vi "applyNewTimes.vi"(8 "error in (no error)":errorcluster, 11 "ScriptEventList in":refnum<class "ScriptEventList.lvclass">) -> (0 "error out":errorcluster, 3 "ScriptEventList out":refnum<class "ScriptEventList.lvclass">)   [LabVIEW 2011, in "Tools.lvlib" / "Scripting.lvlib" / "ScriptEventList.lvclass"]
uses:
  ScriptEventList.lvclass
  ScriptEventList.lvclass/ScriptEventList.ctl
  ScriptEvent.lvclass
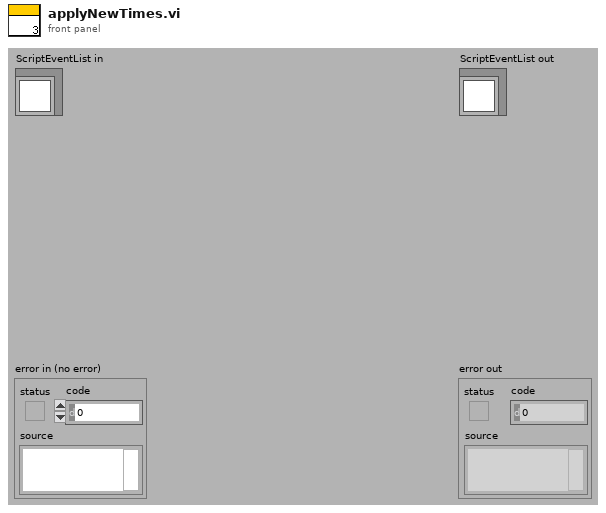
[diagram p1: front panel]
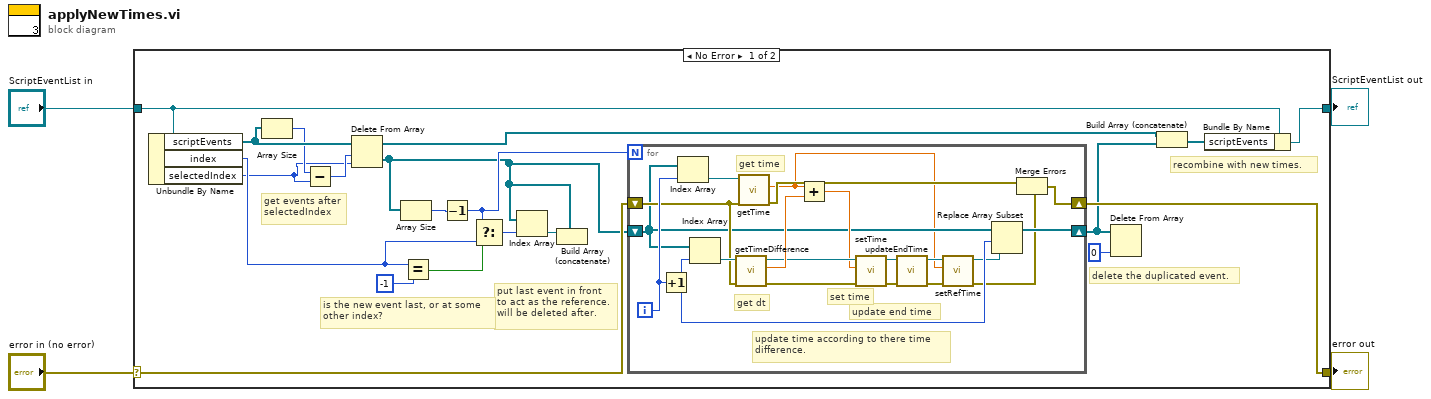
[diagram p0: block diagram]
diagram:
  n1 = case shown="No Error" "error in (no error)" {
    selector: "error in (no error)" -> [w16 w46]
    tunnel: [w10 w46] -> w3
    tunnel: [w11 w45] -> w1
    tunnel: "ScriptEventList in" -> [w12 w45]
    frame No Error {
      # "is the new event last, or at some \nother index?"
      # "recombine with new times."
      # "delete the duplicated event."
      # "put last event in front\nto act as the reference.\nwill be deleted after."
      # "get events after\nselectedIndex"
      n2 = Unbundle By Name(w12) -> ("scriptEvents"=w24:refnum<class "ScriptEvent.lvclass">[], "index"=w8:i32, "selectedIndex"=w7:i32)
      n3 = Array Size(array=w24) -> (size(s)=w9:i32)
      n4 = Subtract(x=w9, y=w7) -> (x-y=w23:i32)
      n5 = Delete From Array(array=w24, length=w23, index=w7) -> (deleted portion=w6:refnum<class "ScriptEvent.lvclass">[], array with subset deleted=w14:refnum<class "ScriptEvent.lvclass">[])
      n6 = Array Size(array=w6) -> (size(s)=w19:i32)
      n7 = Equal?(x=w8, y=-1) -> (x = y?=w22:bool)
      n8 = Decrement(x=w19) -> (x-1=w18:i32)
      n9 = Select(t=w18, s=w22, f=w8) -> (s? t:f=w21:i32)
      n10 = Index Array(array=w6, index=w21) -> (element=w17:refnum<class "ScriptEvent.lvclass">)
      n11 = Build Array (concatenate)(w17, w6) -> ()  [unwired: 1 out]
      n12 = for {
        N: w18 -> [_]
        shift-right: [w34] -> w5
        shift-left: w6 -> [w36]
        shift-right: [w32] -> w10
        shift-left: w16 -> [w41]
        i -> [w44]
        # "update end time"
        # "update time according to there time \ndifference."
        # "get time"
        # "set time"
        # "get dt"
        n13 = Increment(x=w44) -> (x+1=w35:i32)
        n14 = Index Array(array=w36, index=w44) -> (element=w43:refnum<class "ScriptEvent.lvclass">)
        n15 = Index Array(array=w36, index=w35) -> (element=w42:refnum<class "ScriptEvent.lvclass">)
        n16 = call "getTimeDifference.vi"("error in (no error)"=w41, "ScriptEvent.lvclass in"=w42) -> ("error out"=w37:errorcluster, "time difference"=w40:dbl, "ScriptEvent.lvclass out"=w39:refnum<class "ScriptEvent.lvclass">)  [unwired: 7 in]
        n17 = call "getTime.vi"("error in (no error)"=w41, "ScriptEvent.lvclass in"=w43) -> ("error out"=w33:errorcluster, "time"=w27:dbl)  [unwired: 7 in, 1 out]
        n18 = Add(x=w27, y=w40) -> (x+y=w38:dbl)
        n19 = call "setTime.vi"("error in (no error)"=w37, "time"=w38, "ScriptEvent.lvclass in"=w39) -> ("error out"=w31:errorcluster, "ScriptEvent.lvclass out"=w30:refnum<class "ScriptEvent.lvclass">)  [unwired: 7 in]
        n20 = call-dynamic "updateEndTime.vi"("error in (no error)"=w31, "ScriptEvent in"=w30) -> ("error out"=w28:errorcluster, "ScriptEvent out"=w29:refnum<class "ScriptEvent.lvclass">)  [unwired: 8 in]
        n21 = call "setRefTime.vi"("error in (no error)"=w28, "refTime"=w27, "ScriptEvent.lvclass in"=w29) -> ("error out"=w26:errorcluster, "ScriptEvent.lvclass out"=w25:refnum<class "ScriptEvent.lvclass">)  [unwired: 7 in]
        n22 = Replace Array Subset(array=w36, new element=w25, index=w35) -> (w34:refnum<class "ScriptEvent.lvclass">[])
        n23 = Merge Errors(w33, w26) -> (w32:errorcluster)
      }
      n24 = Delete From Array(array=w5, index=0) -> ()  [unwired: 1 in, 2 out]
      n25 = Build Array (concatenate)(w14, w5) -> (w13:refnum<class "ScriptEvent.lvclass">[])
      n26 = Bundle By Name(cluster=w12, "scriptEvents"=w13) -> (w11:refnum<class "ScriptEventList.lvclass">)
    }
    frame Error {
    }
  }
  "error out" <- w3
  "ScriptEventList out" <- w1
